vi "D to Y Conversion.vi"   [LabVIEW 2014, in "NI_EP_Power Quality.lvlib"]
doc: "Converts line voltages to phase voltages. This VI calculates an approximate value for the phase voltage in an unbalanced system because the neutral point is placed at the center of the gravity of the line voltages triangle. When calculating phase voltage values, this VI places the neutral point at the center of gravity of the line voltage triangle, which are the characteristics of a balanced three-phase electrical power system. Thus the phase voltage values this VI returns are approximate values for unbalanced system. You must use this VI before performing power measurement, one-cycle power measurement, and signaling measurement, if the input wiring is line voltage.\n\nThis VI supports measuring single-line and multiple-line systems."
uses:
  <vilib>/addons/Electrical Power/PQ/NI_EP_Power Quality.lvlib
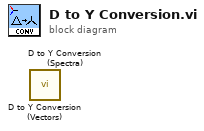
[diagram p0: block diagram]
diagram:
  n1 = call <vilib>:"D to Y Conversion (Vectors).vi"() -> ()  [unwired: 13 in, 3 out]
  n2 = call <vilib>:"D to Y Conversion (Spectra).vi"() -> ()  [unwired: 13 in, 3 out]
